vi "PixyGetData.vi"(11 "I2CDevRef":T2={"DevStatus"={"status"=FALSE, "code"=0, "source"=""}, "Device Address"=0, "Handle"=0, "I2C Bus"=enum."Invalid"} {"Device Address" format="%.0x"}) -> (3 "Data":T1)   [LabVIEW 2017]
uses:
  <vilib>/Rock Robotics/WPI/I2C/WPI_I2CDevRef.ctl
  <vilib>/Rock Robotics/SystemInterfaces/i2clib/i2c_bus.ctl
panel:
  in  "I2CBytesToRead":u8=14
  out "Data Out":u8[](array[numeric]) format="%x"
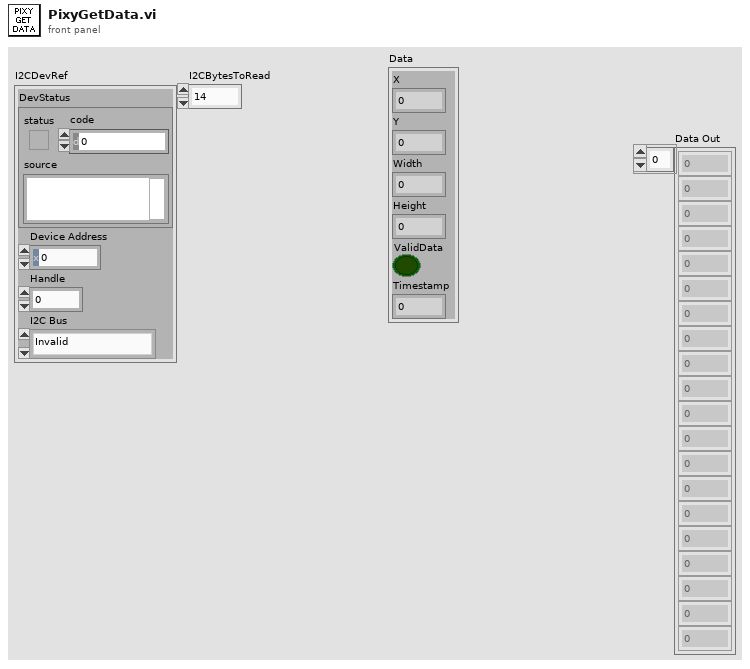
[diagram p1: front panel]
types:
  T1 = cluster{"X":i32, "Y":i32, "Width":i32, "Height":i32, "ValidData":bool, "Timestamp":u32}
  T2 = typedef "WPI_I2CDevRef.ctl" = cluster{"DevStatus":errorcluster, "Device Address":u8, "Handle":i32, "I2C Bus":T3}
  T3 = typedef "i2c_bus.ctl" = enum16{"I2C On-Board", "I2C MXP", "Invalid"}
  T4 = cluster{u16, u16, u16, u16, bool, "millisecond timer value":u32}
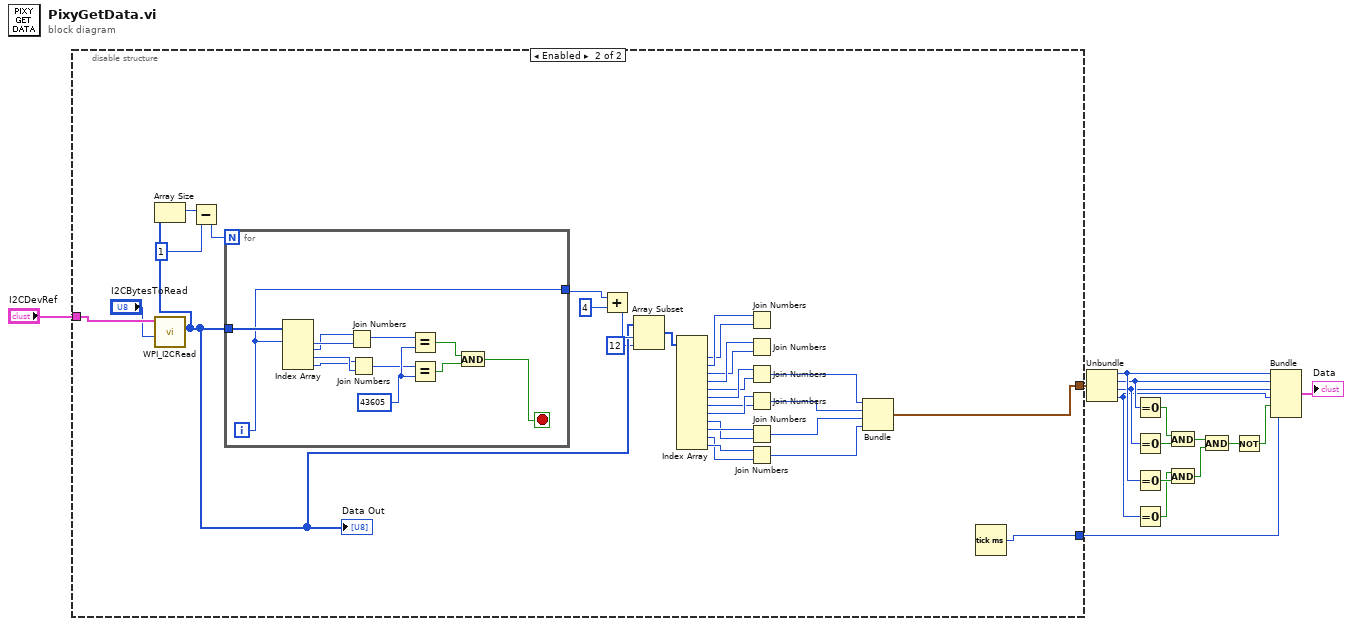
[diagram p0: block diagram]
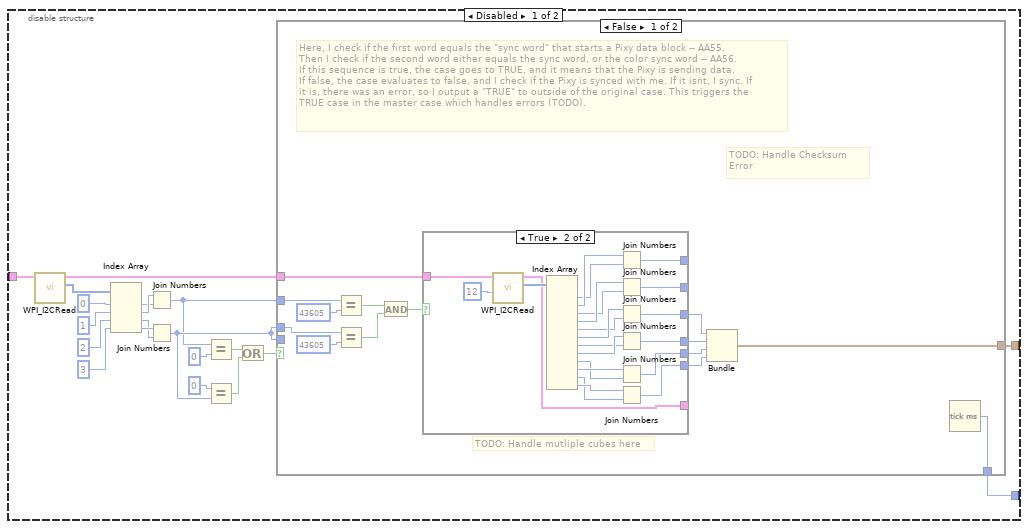
[diagram p2: hidden frame]
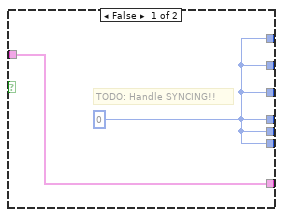
[diagram p3: hidden frame]
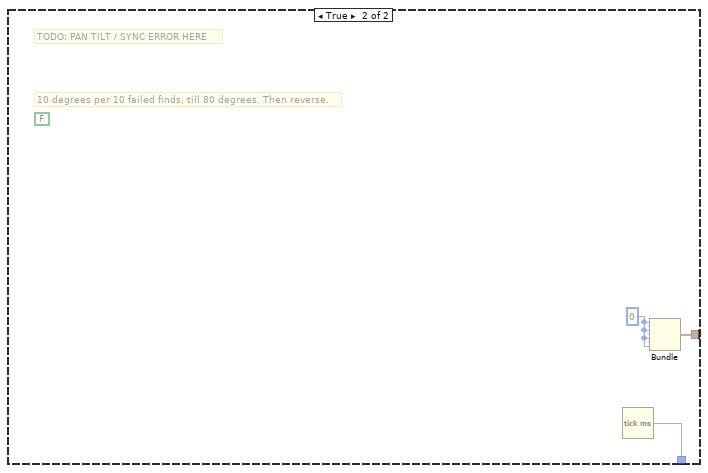
[diagram p4: hidden frame]
diagram:
  n1 = disable-structure shown="Enabled" {
    disable-tunnel: "I2CDevRef" -> [w19 w106]
    disable-tunnel: [w18 w79] -> w8
    disable-tunnel: [w17 w78] -> w1
    frame Disabled {
      n2 = call <vilib>:"WPI_I2CRead.vi"("I2CDevRef"=w19) -> ("Data Out"=w24:u8[], "I2CDevRef"=w34:T2)  [unwired: 8 in, 1 out]
      n3 = Index Array(array=w24, index #1=0 ("index"), index #2=1 ("index"), index #3=2 ("index"), index #4=3 ("index")) -> (element #1=w29:u8, element #2=w30:u8, element #3=w31:u8, element #4=w32:u8)
      n4 = Join Numbers(hi=w30, lo=w29) -> ((hi.lo)=w35:u16)
      n5 = Join Numbers(hi=w32, lo=w31) -> ((hi.lo)=w36:u16)
      n6 = Equal?(x=w35, y=u16 0) -> (x = y?=w22:bool)
      n7 = Equal?(x=u16 0, y=w36) -> (x = y?=w23:bool)
      n8 = Or(x=w22, y=w23) -> (x .or. y?=w33:bool)
      n9 = case shown="False" w33 {
        tunnel: w34 -> [w47 _]
        tunnel: w35 -> [w46 _]
        tunnel: w36 -> [w45 _]
        tunnel: w36 -> [_ _]
        tunnel: [w38 w76] -> w18
        tunnel: [w37 w75] -> w17
        frame False {
          # "TODO: Handle Checksum \nError"
          # "TODO: Handle mutliple cubes here"
          # "Here, I check if the first word equals the \"sync word\" that starts a Pixy data block -- AA55. \nThen I check if the second word either equals the sync word, or the color sync word -- AA56.\nIf this sequence is true, the case goes to TRUE, and it means that the Pixy is sending data.\nIf false, the case evaluates to false, and I check if the Pixy is synced with me. If it isnt, I sync. If\nit is, there was an error, so I output a \"TRUE\" to outside of the original case. This triggers the \nTRUE case in the master case which handles errors (TODO)."
          n10 = Equal?(x=w46, y=u16 43605) -> (x = y?=w50:bool)
          n11 = Equal?(x=w45, y=u16 43605) -> (x = y?=w44:bool)
          n12 = And(x=w50, y=w44) -> (x .and. y?=w43:bool)
          n13 = case shown="True" w43 {
            tunnel: w47 -> [w51 w74]
            tunnel: [w52 w60] -> w39
            tunnel: [w52 w59] -> w40
            tunnel: [w52 w58] -> w41
            tunnel: [w52 w57] -> w42
            tunnel: [w52 w56] -> _
            tunnel: [w52 w55] -> _
            tunnel: [w51 w53] -> _
            frame False {
              w52 = 0
              # "TODO: Handle SYNCING!!"
            }
            frame True {
              n14 = call <vilib>:"WPI_I2CRead.vi"("I2CBytesToRead"=u8 12, "I2CDevRef"=w74) -> ("Data Out"=w54:u8[], "I2CDevRef"=w53:T2)  [unwired: 7 in, 1 out]
              n15 = Index Array(array=w54) -> (element #1=w61:u8, element #2=w62:u8, element #3=w63:u8, element #4=w64:u8, element #5=w65:u8, element #6=w66:u8, element #7=w67:u8, element #8=w68:u8, element #9=w69:u8, element #10=w70:u8, element #11=w71:u8, element #12=w72:u8)  [unwired: 12 in]
              n16 = Join Numbers(hi=w62, lo=w61) -> ((hi.lo)=w55:u16)
              n17 = Join Numbers(hi=w64, lo=w63) -> ((hi.lo)=w56:u16)
              n18 = Join Numbers(hi=w66, lo=w65) -> ((hi.lo)=w57:u16)
              n19 = Join Numbers(hi=w68, lo=w67) -> ((hi.lo)=w58:u16)
              n20 = Join Numbers(hi=w70, lo=w69) -> ((hi.lo)=w59:u16)
              n21 = Join Numbers(hi=w72, lo=w71) -> ((hi.lo)=w60:u16)
            }
          }
          n22 = Bundle(w42, w41, w40, w39) -> (w38:cluster{i32, i32, i32, i32})  [unwired: 1 in]
          n23 = Tick Count (ms)() -> (millisecond timer value=w37:u32)
        }
        frame True {
          (unwired) FALSE
          w77 = 0
          # "10 degrees per 10 failed finds, till 80 degrees. Then reverse."
          # "TODO: PAN TILT / SYNC ERROR HERE"
          n24 = Tick Count (ms)() -> (millisecond timer value=w75:u32)
          n25 = Bundle(w77, w77, w77, w77) -> (w76:cluster{i32, i32, i32, i32})  [unwired: 1 in]
        }
      }
    }
    frame Enabled {
      n26 = call <vilib>:"WPI_I2CRead.vi"("I2CBytesToRead"="I2CBytesToRead", "I2CDevRef"=w106) -> ("Data Out"=w86:u8[])  [unwired: 7 in, 2 out]
      "Data Out" <- w86
      n27 = Array Size(array=w86) -> (size(s)=w104:i32)
      n28 = Subtract(x=w104, y=1) -> (x-y=w102:i32)
      n29 = for {
        N: w102 -> [_]
        tunnel: w86 -> [w118]
        tunnel: [w107] -> w89
        i -> [w107]
        stop <- w108 stop-if-true
        w112 = 43605 ("y")
        n30 = Index Array(array=w118, index #1=w107) -> (element #1=w117:u8, element #2=w116:u8, element #3=w115:u8, element #4=w114:u8)  [unwired: 3 in]
        n31 = Join Numbers(hi=w116, lo=w117) -> ((hi.lo)=w113:u16)
        n32 = Join Numbers(hi=w114, lo=w115) -> ((hi.lo)=w111:u16)
        n33 = Equal?(x=w113, y=w112) -> (x = y?=w110:bool)
        n34 = Equal?(x=w111, y=w112) -> (x = y?=w109:bool)
        n35 = And(x=w110, y=w109) -> (x .and. y?=w108:bool)
      }
      n36 = Add(x=w89, y=4) -> (x+y=w87:i32)
      n37 = Array Subset(array=w86, index=w87, length=12) -> (w84:u8[])
      n38 = Index Array(array=w84) -> (element #1=w90:u8, element #2=w91:u8, element #3=w92:u8, element #4=w93:u8, element #5=w94:u8, element #6=w95:u8, element #7=w96:u8, element #8=w97:u8, element #9=w98:u8, element #10=w99:u8, element #11=w100:u8, element #12=w101:u8)  [unwired: 12 in]
      n39 = Join Numbers(hi=w91, lo=w90) -> ()  [unwired: 1 out]
      n40 = Join Numbers(hi=w93, lo=w92) -> ()  [unwired: 1 out]
      n41 = Join Numbers(hi=w95, lo=w94) -> ((hi.lo)=w83:u16)
      n42 = Join Numbers(hi=w97, lo=w96) -> ((hi.lo)=w82:u16)
      n43 = Join Numbers(hi=w99, lo=w98) -> ((hi.lo)=w81:u16)
      n44 = Join Numbers(hi=w101, lo=w100) -> ((hi.lo)=w80:u16)
      n45 = Bundle(w83, w82, w81, w80) -> (w79:cluster{u16, u16, u16, u16})  [unwired: 1 in]
      n46 = Tick Count (ms)() -> (millisecond timer value=w78:u32)
    }
  }
  n47 = Unbundle(w8) -> (w7:u16, w6:u16, w5:u16, w4:u16)
  n48 = Equal To 0?(x=w6) -> (x = 0?=w15:bool)
  n49 = Equal To 0?(x=w5) -> (x = 0?=w10:bool)
  n50 = Equal To 0?(x=w7) -> (x = 0?=w12:bool)
  n51 = Equal To 0?(x=w4) -> (x = 0?=w11:bool)
  n52 = And(x=w15, y=w10) -> (x .and. y?=w13:bool)
  n53 = And(x=w11, y=w12) -> (x .and. y?=w14:bool)
  n54 = And(x=w13, y=w14) -> (x .and. y?=w16:bool)
  n55 = Not(x=w16) -> (.not. x?=w3:bool)
  n56 = Bundle(w7, w6, w5, w4, w3, "millisecond timer value"=w1) -> (→"Data":T4)  [unwired: 1 in]
